vi "SATPdll_d.vi"(5 "dll_path_in":path, 8 "error in (no error)":errorcluster, 9 "Component Molar Fractions":dbl[](array[numeric])=[1.0, 0.0, 0.0, 0.0, 0.0, 0.0, 0.0, 0.0, 0.0, 0.0, 0.0, 0.0, 0.0, 0.0, 0.0, 0.0, 0.0, 0.0, 0.0, 0.0], 10 "i":i32, 11 "Press (kPa)":dbl=30.0) -> (0 "error out":errorcluster, 3 "pdataout":dbl[](array[numeric]), 4 "dll_path_out":path)   [LabVIEW 2017]
doc: "Calculate saturated liquid and vapor states given pressure and the composition of one phase\n\n inputs:\n p--pressure [kPa]\n x--composition [array of mol frac] (phase specified by kph)\n kph--phase flag: 1 = input x is liquid composition\n 2 = input x is vapor composition\n\n outputs:\n t--temperature [K]\n rhol--molar density [mol/L] of saturated liquid\n rhov--molar density [mol/L] of saturated vapor\n xliq--liquid phase composition [array of mol frac]\n xvap--vapor phase composition [array of mol frac]\n ierr--error flag: 0 = successful\n 4 = P < 0\n 8 = x out of range\n 12 = P and x out of range\n 140 = CRITP did not converge\n 141 = P > Pcrit\n 142 = TPRHO-liquid did not converge (pure fluid)\n 143 = TPRHO-vapor did not converge (pure fluid)\n 144 = pure fluid iteration did not converge\n following 3 error codes are advisory--iteration will either\n converge on later guess or error out (ierr = 148)\n -144 = Raoult's law (mixture intial guess) did not converge\n -145 = TPRHO did not converge for parent ph (mix)\n -146 = TPRHO did not converge for incipient (mix)\n -147 = composition iteration did not converge\n 148 = mixture iteration did not converge\n herr--error string if ierr<>0 (character*255))t"
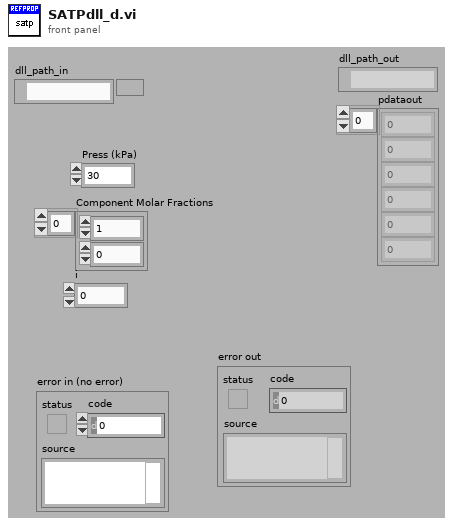
[diagram p1: front panel]
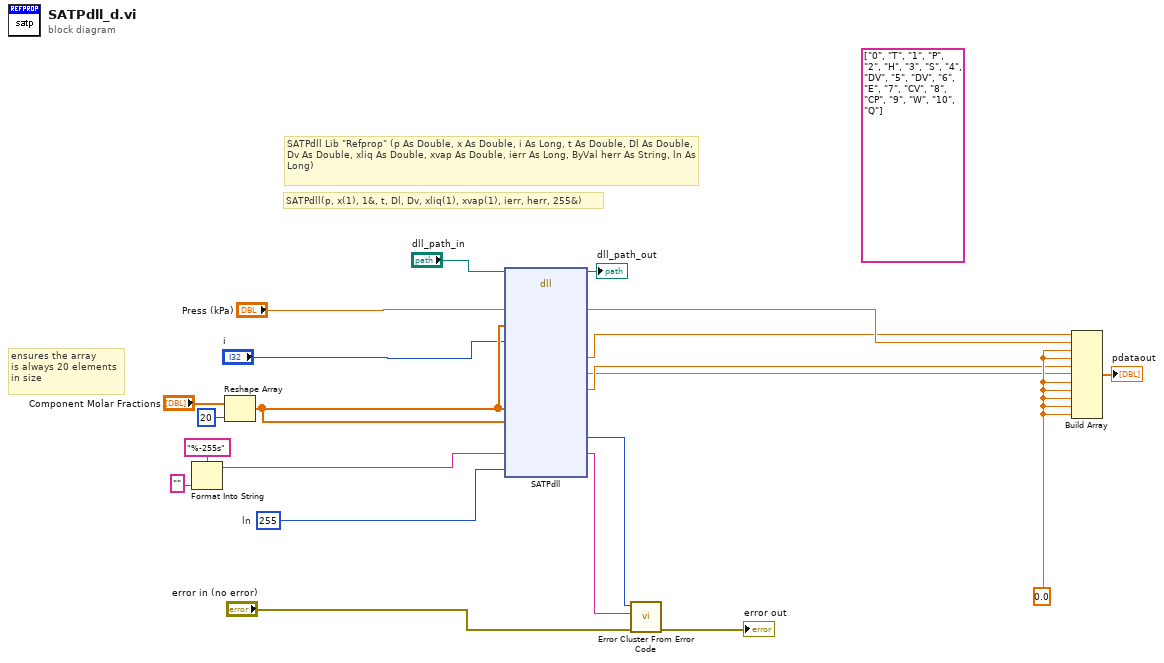
[diagram p0: block diagram]
diagram:
  (unwired) string[][] [["0", "T"], ["1", "P"], ["2", "H"], ["3", "S"], ["4", "DV"], ["5", "DV"], ["6", "E"], ["7", "CV"], ["8", "CP"], ["9", "W"], ["10", "Q"]] ("数组")
  w6 = 0.0 ("h")
  w11 = 255  # ln
  # "SATPdll Lib \"Refprop\" (p As Double, x As Double, i As Long, t As Double, Dl As Double, Dv As Double, xliq As Double, xvap As Double, ierr As Long, ByVal herr As String, ln As Long)"
  # "SATPdll(p, x(1), 1&, t, Dl, Dv, xliq(1), xvap(1), ierr, herr, 255&)"
  # "ensures the array\nis always 20 elements\nin size"
  n1 = Format Into String(format string="%-255s", "") -> (resulting string=w10:string)  [unwired: 2 in, 1 out]
  n2 = Reshape Array("Component Molar Fractions", 20 ("dimension size")) -> (w17:dbl[])
  n3 = dll-call lib="refprop.DLL" fn="SATPdll" label="satPDLL"(path in="dll_path_in", "p"="Press (kPa)", "x"=w17, "i"="i", "xliq"=w17, "xvap"=w17, "herr"=w10, "ln"=w11) -> (path out=→"dll_path_out":path, "p"=w7:dbl, "t"=w5:dbl, "Dl"=w3:dbl, "Dv"=w4:dbl, "ierr"=w12:i32, "herr"=w13:string)  [unwired: 12 in, 1 out]
  n4 = call <vilib>:"Error Cluster From Error Code.vi"("error in (no error)"="error in (no error)", "error message (\"\")"=w13, "error code (0)"=w12) -> ("error out"=→"error out":errorcluster)  [unwired: 6 in]
  n5 = Build Array(w5, w7, w6, w6, w4, w3, w6, w6, w6, w6, w6) -> (→"pdataout":dbl[])
